vi "Build_Header_Python.vi"(9 "ERD Number Array":string[](array[string]), 10 "ERD Name Array In":string[](array[string]), 11 "ERD_Data_Bound":T1) -> (3 "ERD Name Array out":string[][](array[string]))   [LabVIEW 2021]
uses:
  Controles/ERD_Data_Boundled.ctl
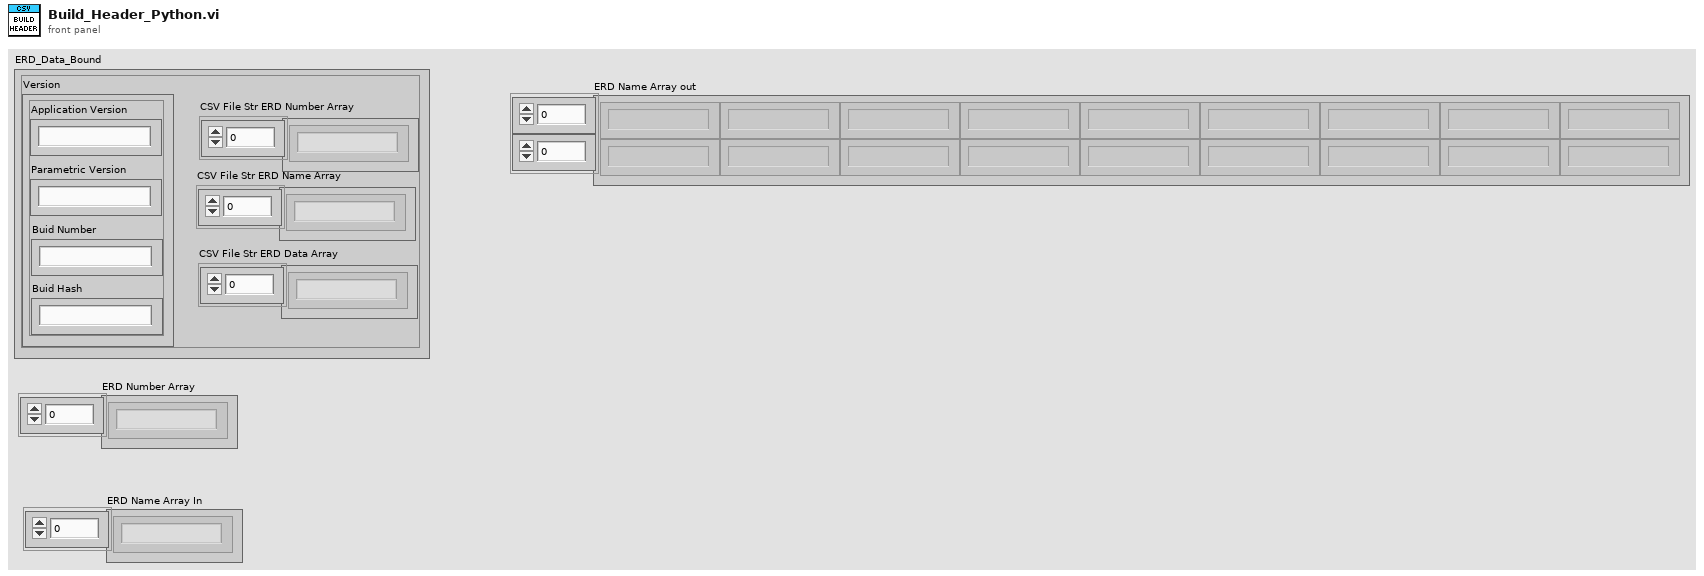
[diagram p1: front panel]
types:
  T1 = typedef "ERD_Data_Boundled.ctl" = cluster{"Version":cluster{"Application Version":string, "Parametric Version":string, "Buid Number":string, "Buid Hash":string}, "CSV File Str ERD Name Array":string[], "CSV File Str ERD Number Array":string[], "CSV File Str ERD Data Array":string[]}
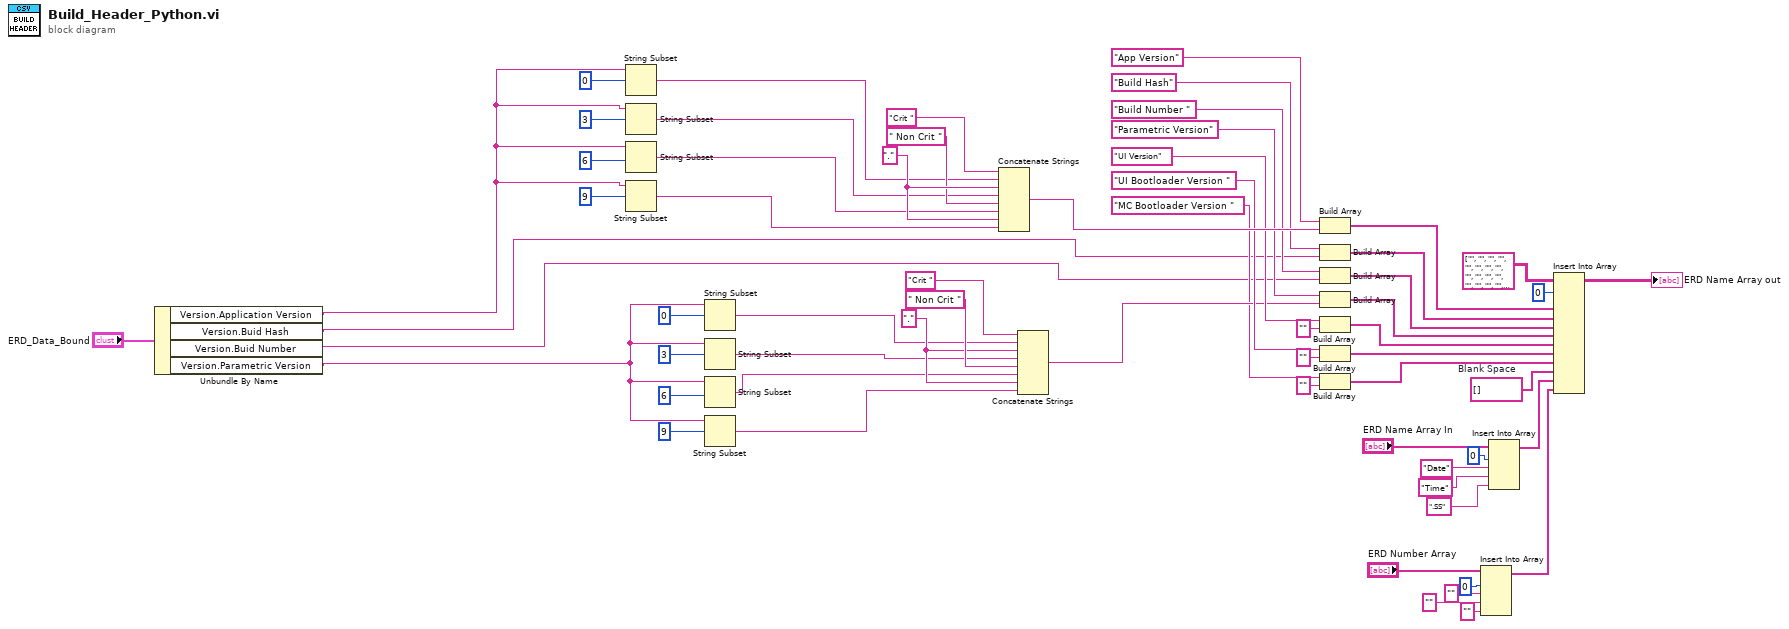
[diagram p0: block diagram]
diagram:
  w33 = string[] []  # Blank Space
  w57 = "." ("element")
  w62 = "." ("element")
  n1 = Unbundle By Name("ERD_Data_Bound") -> ("Version.Application Version"=w13:string, "Version.Buid Hash"=w12:string, "Version.Buid Number"=w11:string, "Version.Parametric Version"=w10:string)
  n2 = String Subset(string=w13, offset (0)=0 ("length (rest)")) -> (substring=w26:string)  [unwired: 1 in]
  n3 = String Subset(string=w13, offset (0)=3 ("length (rest)")) -> (substring=w25:string)  [unwired: 1 in]
  n4 = String Subset(string=w13, offset (0)=6) -> (substring=w24:string)  [unwired: 1 in]
  n5 = String Subset(string=w13, offset (0)=9) -> (substring=w23:string)  [unwired: 1 in]
  n6 = String Subset(string=w10, offset (0)=0 ("length (rest)")) -> (substring=w18:string)  [unwired: 1 in]
  n7 = String Subset(string=w10, offset (0)=3 ("length (rest)")) -> (substring=w17:string)  [unwired: 1 in]
  n8 = String Subset(string=w10, offset (0)=6) -> (substring=w16:string)  [unwired: 1 in]
  n9 = String Subset(string=w10, offset (0)=9) -> (substring=w15:string)  [unwired: 1 in]
  n10 = Concatenate Strings("Crit " ("element"), w26, w62, w25, " Non Crit " ("element"), w24, w62, w23) -> (w53:string)
  n11 = Concatenate Strings("Crit " ("element"), w18, w57, w17, " Non Crit " ("element"), w16, w57, w15) -> (w37:string)
  n12 = Build Array("App Version" ("new element/subarray"), w53) -> (w55:string[])
  n13 = Build Array("Build Hash" ("new element/subarray"), w12) -> (w51:string[])
  n14 = Build Array("Build Number " ("new element/subarray"), w11) -> (w49:string[])
  n15 = Build Array("Parametric Version" ("new element/subarray"), w37) -> (w48:string[])
  n16 = Build Array("UI Version" ("new element/subarray"), "" ("element")) -> (w47:string[])
  n17 = Build Array("UI Bootloader Version " ("new element/subarray"), "" ("element")) -> (w36:string[])
  n18 = Build Array("MC Bootloader Version " ("new element/subarray"), "" ("element")) -> (w31:string[])
  n19 = Insert Into Array(array="ERD Number Array", index=0, new element #1="" ("new element/subarray"), new element #2="" ("new element/subarray"), new element #3="" ("new element/subarray")) -> (w1:string[])
  n20 = Insert Into Array(array="ERD Name Array In", index=0, new element #1="Date", new element #2="Time", new element #3=".SS" ("new element/subarray")) -> (w32:string[])
  n21 = Insert Into Array(array=string[][] [["", "", "", "", "", "", "", "", "", "", "", "", "", "", "", "", "", "", "", "", "", "", "", "", "", "", "", "", "", "", "", "", "", "", "", "", "", "", "", "", "0"]] ("Array Ini"), index (row)=0, new element #1=w55, new element #2=w51, new element #3=w49, new element #4=w48, new element #5=w47, new element #6=w36, new element #7=w31, new element #8=w33, new element #9=w32, new element #10=w1) -> (→"ERD Name Array out":string[][])  [unwired: 1 in]
